vi "Igor replace bad symbols.vi"(11 "names":string[](array[string])) -> (3 "Igor Igor names":string[](array[string]))   [LabVIEW 2025]
panel:
  # "Igor has certain rules for the wave name; \n1.  Only numbers, alphabet letters and underscore (_) are allowed.\n2.  Wave name must start with an alphabet letter."
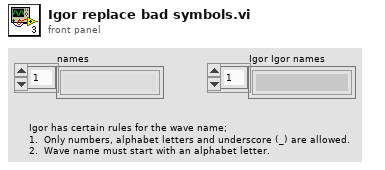
[diagram p1: front panel]
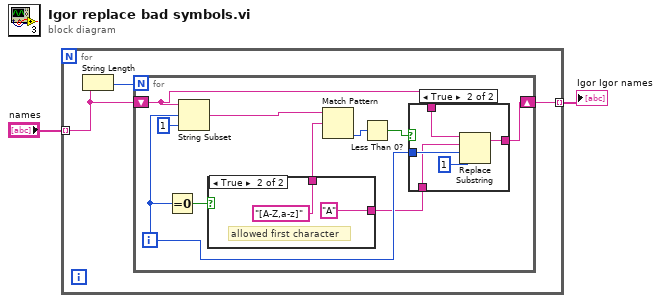
[diagram p0: block diagram]
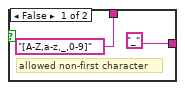
[diagram p2: hidden frame]
diagram:
  n1 = for {
    tunnel: "names" -> [w4] mode=indexing
    tunnel: [w3] -> w1 mode=indexing
    n2 = String Length(string=w4) -> (length=w5:i32)
    n3 = for {
      N: w5 -> [_]
      shift-right: [w9] -> w3
      shift-left: w4 -> [w11]
      i -> [w10]
      n4 = Equal To 0?(x=w10) -> (x = 0?=w13:bool)
      n5 = String Subset(string=w11, offset (0)=w10, length (rest)=1 ("length (rest)")) -> (substring=w14:string)
      n6 = case shown="True" w13 {
        tunnel: ["[A-Z,a-z,_,0-9]" ("regular expression") "[A-Z,a-z]" ("regular expression")] -> w12
        tunnel: ["_" ("substring (\"\")") "A" ("substring (\"\")")] -> w6
        frame False {
          # "allowed non-first character"
        }
        frame True {
          # "allowed first character"
        }
      }
      n7 = Match Pattern(string=w14, regular expression=w12) -> (offset past match=w8:i32)  [unwired: 1 in, 3 out]
      n8 = Less Than 0?(x=w8) -> (x < 0?=w7:bool)
      n9 = case shown="True" w7 {
        tunnel: w11 -> [w20 w25]
        tunnel: w10 -> [_ w24]
        tunnel: [w20 w22] -> w9
        tunnel: w6 -> [_ w21]
        frame False {
        }
        frame True {
          n10 = Replace Substring(2:1 ("length (len. of substring)"), 3:w24, 4:w21, 5:w25) -> (1:w22:string)  [unwired: 1 out]
        }
      }
    }
  }
  "Igor Igor names" <- w1
